vi "x3_.vi"() -> ()   [LabVIEW 2014]
panel:
  in  "x3_":dbl
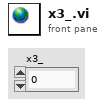
[diagram p1: front panel]
diagram:
